vi "4_lab.vi"() -> ()   [LabVIEW 2013]
panel:
  out "Message":string
  in  "TMax":dbl
  in  "TMin":dbl
  out "Indicator":bool
  out "Output":dbl
  out "Waveform Chart":dbl(graph)
  out "t":dbl(slide) scale=-50.0..50.0
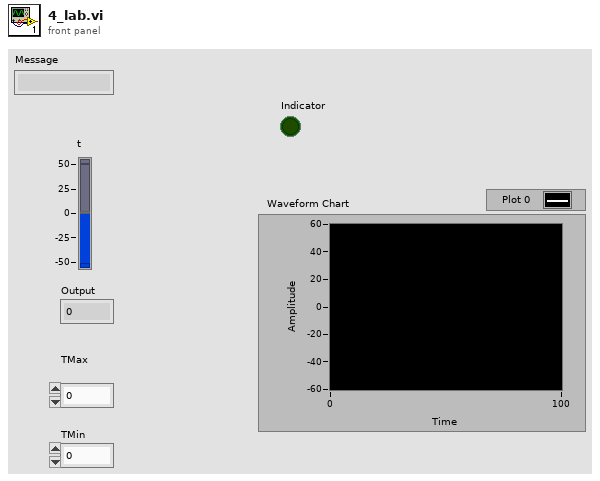
[diagram p1: front panel]
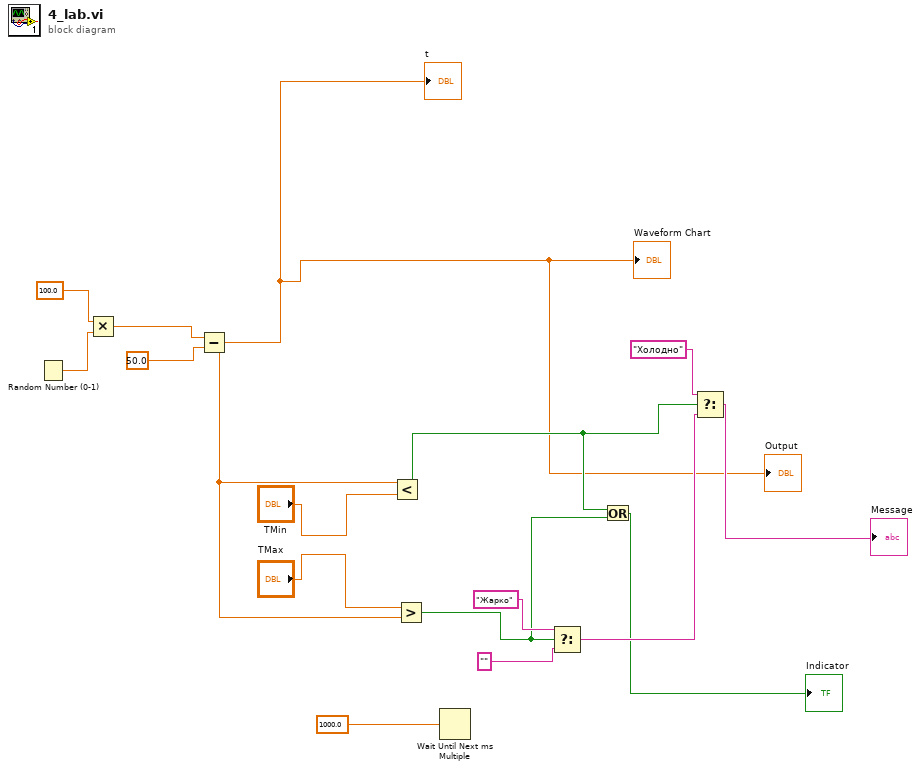
[diagram p0: block diagram]
diagram:
  n1 = Random Number (0-1)() -> (number: 0 to 1=w16:dbl)
  n2 = Multiply(x=100.0 ("Numeric 2"), y=w16) -> (x*y=w14:dbl)
  n3 = Subtract(x=w14, y=50.0 ("Numeric 2")) -> (x-y=w1:dbl)
  "t" <- w1
  "Waveform Chart" <- w1
  "Output" <- w1
  n4 = Less?(x=w1, y="TMin") -> (x < y?=w4:bool)
  n5 = Greater?(x="TMax", y=w1) -> (0:w3:bool)
  n6 = Wait Until Next ms Multiple(millisecond multiple=1000.0 ("Numeric 2")) -> ()  [unwired: 1 out]
  n7 = Select(t="Жарко", s=w3, f="") -> (s? t:f=w9:string)
  n8 = Or(x=w4, y=w3) -> (x .or. y?=→"Indicator":bool)
  n9 = Select(t="Холодно", s=w4, f=w9) -> (s? t:f=→"Message":string)
